vi "Write FXPIL.vi"(8 "error in (no error)":errorcluster, 10 "FXPIL":i32, 11 "Channel_FXP in":refnum<class "Channel_FXP.lvclass">) -> (0 "error out":errorcluster, 3 "Channel_FXP out":refnum<class "Channel_FXP.lvclass">)   [LabVIEW 2013, in "Channel_FXP.lvclass"]
uses:
  Channel_FXP.lvclass
  Channel_FXP.lvclass/Channel_FXP.ctl
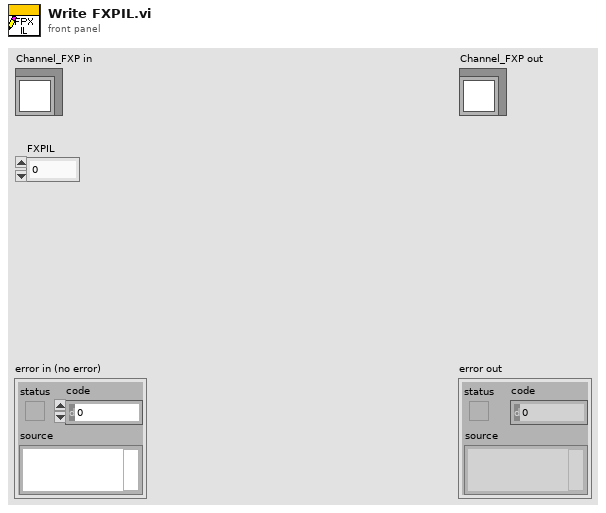
[diagram p1: front panel]
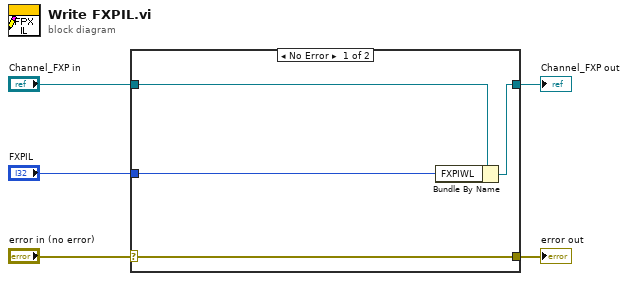
[diagram p0: block diagram]
diagram:
  n1 = case shown="No Error" "error in (no error)" {
    selector: "error in (no error)" -> [w9 w10]
    tunnel: [w9 w10] -> w4
    tunnel: [w7 w11] -> w2
    tunnel: "Channel_FXP in" -> [w8 w11]
    tunnel: "FXPIL" -> [w6 _]
    frame No Error {
      n2 = Bundle By Name(cluster=w8, "FXPIWL"=w6) -> (w7:refnum<class "Channel_FXP.lvclass">)
    }
    frame Error {
    }
  }
  "error out" <- w4
  "Channel_FXP out" <- w2
